vi "ControlAcceleration.vi"(1 "Backward Acceleration (p/s)":dbl, 2 "Raw":dbl, 3 "Forward Acceleration (p/s)":dbl) -> (0 "Controlled":dbl)   [LabVIEW 2018]
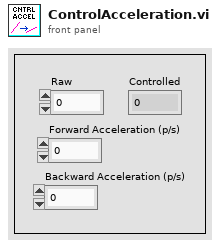
[diagram p1: front panel]
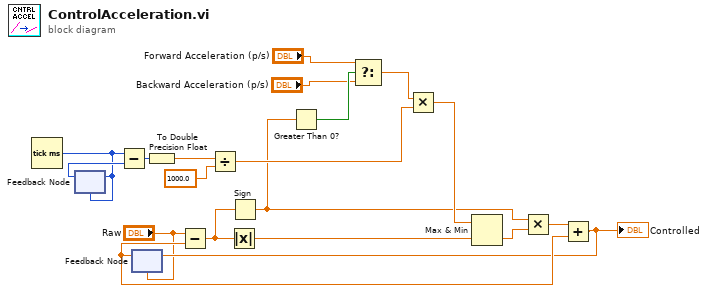
[diagram p0: block diagram]
diagram:
  n1 = Tick Count (ms)() -> (millisecond timer value=w13:u32)
  n2 = feedback-in #1(w13) -> ()
  n3 = feedback #1(w13) -> (w14:u32)
  n4 = Subtract(x=w13, y=w14) -> (x-y=w12:u32)
  n5 = feedback #2("Raw") -> (w15:dbl)
  n6 = To Double Precision Float(number=w12) -> (double precision float=w10:dbl)
  n7 = Subtract(x="Raw", y=w15) -> (x-y=w19:dbl)
  n8 = Divide(x=w10, y=1000.0) -> (x/y=w9:dbl)
  n9 = Absolute Value(x=w19) -> (abs(x)=w18:dbl)
  n10 = Sign(1:w19) -> (0:w4:dbl)
  n11 = Greater Than 0?(x=w4) -> (x > 0?=w3:bool)
  n12 = Select(t="Forward Acceleration (p/s)", s=w3, f="Backward Acceleration (p/s)") -> (s? t:f=w5:dbl)
  n13 = Multiply(x=w5, y=w9) -> (x*y=w11:dbl)
  n14 = Max & Min(x=w11, y=w18) -> (min(x,y)=w17:dbl)  [unwired: 1 out]
  n15 = Multiply(x=w4, y=w17) -> (x*y=w16:dbl)
  n16 = Add(x=w16, y=w15) -> (x+y=w7:dbl)
  "Controlled" <- w7
  n17 = feedback-in #2(w7) -> ()
